vi "pcfs_generate_stage_positions.vi"(5 "travel_min (mm)":dbl, 6 "custom_positions":dbl[](array[numeric]), 7 "travel_max (mm)":dbl, 8 "error in (no error)":errorcluster, 9 "custom_trajectory":bool, 10 "pcfs_settings":T1, 11 "scan_panel in":refnum<class "pcfs.lvclass">) -> (0 "error out":errorcluster, 1 "Dither Movement":dbl, 2 "Positions (mm)":dbl[](array[numeric]), 3 "scan_panel out":refnum<class "pcfs.lvclass">, 4 "Dither_Speed":dbl)   [LabVIEW 2015, in "pcfs.lvclass"]
uses:
  pcfs.lvclass
  pcfs_position_settings.ctl
  <vilib>/Analysis/1siggen.llb/Ramp Pattern by Delta.vi
  <vilib>/Analysis/NI_AALBase.lvlib
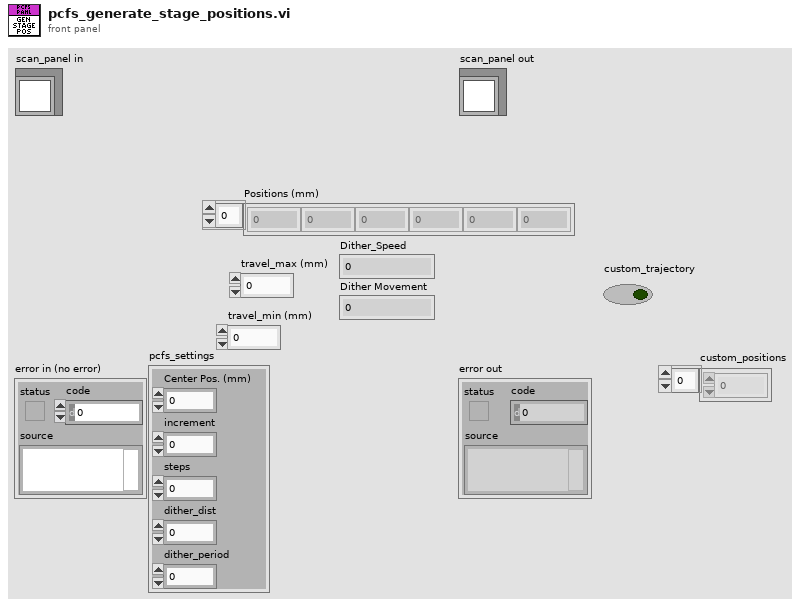
[diagram p1: front panel]
types:
  T1 = typedef "pcfs_position_settings.ctl" = cluster{"Center Pos. (mm)":dbl, "increment":dbl, "steps":dbl, "dither_dist":dbl, "dither_period":dbl}
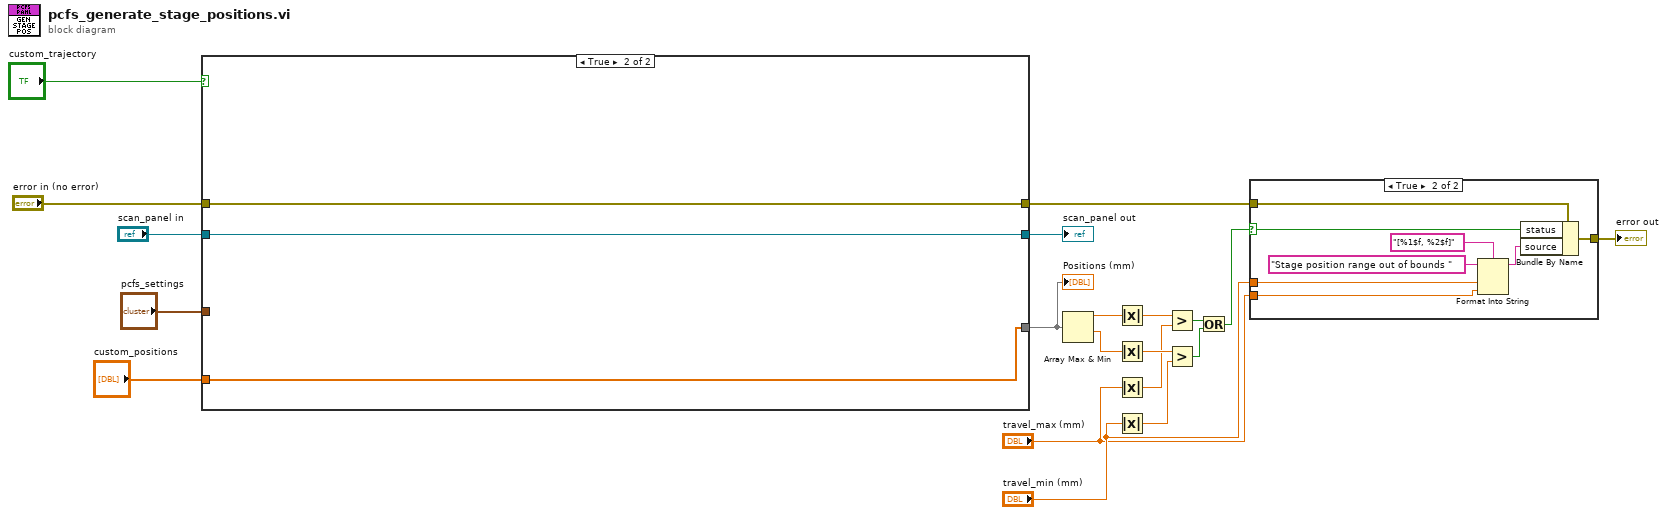
[diagram p0: block diagram]
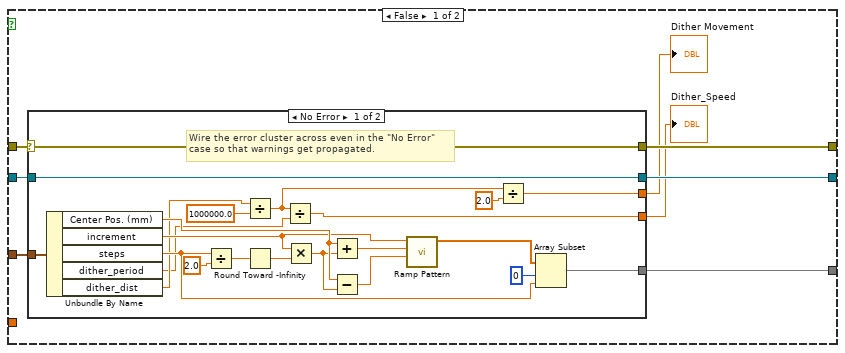
[diagram p2: hidden frame]
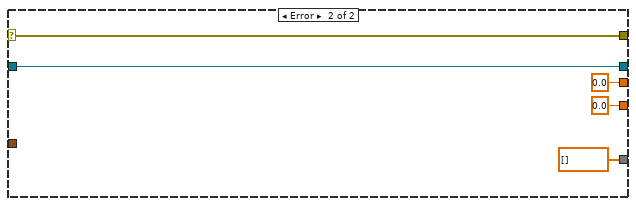
[diagram p3: hidden frame]
diagram:
  n1 = case shown="True" "custom_trajectory" {
    tunnel: "error in (no error)" -> [w28 w57]
    tunnel: "scan_panel in" -> [w27 w58]
    tunnel: [w26 w58] -> w18
    tunnel: [w25 w56] -> w17
    tunnel: [w24 w57] -> w10
    tunnel: "pcfs_settings" -> [w23 _]
    tunnel: "custom_positions" -> [_ w56]
    frame False {
      n2 = case shown="No Error" w28 {
        selector: w28 -> [w49 w55]
        tunnel: [w49 w55] -> w24
        tunnel: [w50 w54] -> w26
        tunnel: w27 -> [w50 w54]
        tunnel: w23 -> [w48 _]
        tunnel: [w36 dbl[] [] ("Ramp Pattern")] -> w25
        tunnel: [w32 0.0] -> w22
        tunnel: [w29 0.0] -> w21
        frame No Error {
          # "Wire the error cluster across even in the \"No Error\"\ncase so that warnings get propagated."
          n3 = Unbundle By Name(w48) -> ("Center Pos. (mm)"=w46:dbl, "increment"=w40:dbl, "steps"=w38:dbl, "dither_period"=w33:dbl, "dither_dist"=w34:dbl)
          n4 = Divide(x=w38, y=2.0) -> (x/y=w42:dbl)
          n5 = Divide(x=w34, y=1000000.0) -> (x/y=w31:dbl)
          n6 = Round Toward -Infinity(1:w42) -> (0:w41:dbl)
          n7 = Divide(x=w31, y=w33) -> (x/y=w32:dbl)
          n8 = Multiply(x=w40, y=w41) -> (x*y=w45:dbl)
          n9 = Add(x=w46, y=w45) -> (x+y=w44:dbl)
          n10 = Subtract(x=w46, y=w45) -> (x-y=w43:dbl)
          n11 = call-poly <vilib>:"Ramp Pattern.vi"("start"=w43, "end"=w44, "delta"=w40) -> ("Ramp Pattern"=w37:dbl[])  [unwired: 6 in, 2 out]
          n12 = Divide(x=w31, y=2.0) -> (x/y=w29:dbl)
          n13 = Array Subset(array=w37, index=0, length=w38) -> (w36:dbl[])
        }
        frame Error {
        }
      }
      "Dither_Speed" <- w22
      "Dither Movement" <- w21
    }
    frame True {
    }
  }
  "scan_panel out" <- w18
  "Positions (mm)" <- w17
  n14 = Array Max & Min(array=w17) -> (max value=w16:dbl, min value=w15:dbl)  [unwired: 2 out]
  n15 = Absolute Value(x=w16) -> (abs(x)=w14:dbl)
  n16 = Absolute Value(x=w15) -> (abs(x)=w13:dbl)
  n17 = Absolute Value(x="travel_max (mm)") -> (abs(x)=w6:dbl)
  n18 = Absolute Value(x="travel_min (mm)") -> (abs(x)=w7:dbl)
  n19 = Greater?(x=w14, y=w6) -> (0:w12:bool)
  n20 = Greater?(x=w13, y=w7) -> (0:w11:bool)
  n21 = Or(x=w12, y=w11) -> (x .or. y?=w9:bool)
  n22 = case shown="True" w9 {
    selector: w9 -> [_ w66]
    tunnel: w10 -> [w59 w67]
    tunnel: [w59 w65] -> w8
    tunnel: "travel_min (mm)" -> [_ w63]
    tunnel: "travel_max (mm)" -> [_ w62]
    frame False {
    }
    frame True {
      n23 = Format Into String(format string="[%1$f, %2$f]", initial string="Stage position range out of bounds " ("source"), w63, w62) -> (resulting string=w61:string)  [unwired: 1 in, 1 out]
      n24 = Bundle By Name(cluster=w67, "status"=w66, "source"=w61) -> (w65:errorcluster)
    }
  }
  "error out" <- w8
